vi "Format File Property.vi"(8 "错误输入":cluster{"状态":bool, "代码":i32, "源":string}, 9 "文件属性值":string, 10 "文件属性名称":string, 11 "字符串输入":string) -> (0 "错误输出":cluster{"状态":bool, "代码":i32, "源":string}, 3 "字符串输出":string)   [LabVIEW 2012]
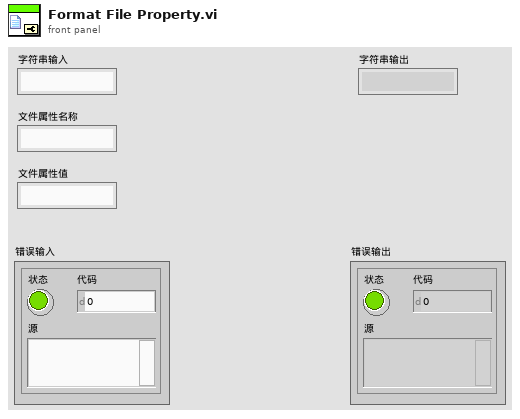
[diagram p1: front panel]
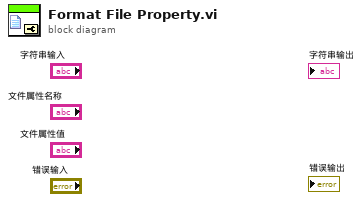
[diagram p0: block diagram]
diagram:
